vi "Server_Main Stop.vi"(8 "error in":errorcluster) -> (0 "error out":errorcluster)   [LabVIEW 2018, in "Cloud Server.lvlib"]
uses:
  Cloud Server.lvlib
  Data Def/Server_Main Loop Queue Data.ctl
  Data Def/Server_Main Loop State.ctl
  Data Def/Server_Server Write Queue Data.ctl
  Data Def/Server_FGV Method.ctl
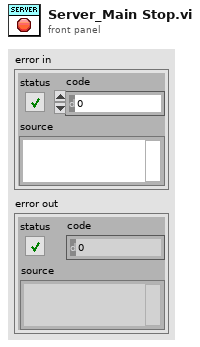
[diagram p1: front panel]
types:
  T1 = typedef "Cloud Server.lvlib/Server_Server Write Queue Data.ctl" = cluster{"connection ID":refnum<k5>, "Meta Data":string, "Data":variant}
  T2 = typedef "Cloud Server.lvlib/Server_Main Loop Queue Data.ctl" = cluster{"Main Loop State":T3, "Data":variant}
  T3 = typedef "Cloud Server.lvlib/Server_Main Loop State.ctl" = enum16{"Detect", "Save", "Training", "Refresh User Name", "Stop"}
  T4 = typedef "Cloud Server.lvlib/Server_FGV Method.ctl" = enum16{"Get", "Put"}
  T5 = typedef "Cloud Server.lvlib/Server_Main Data.ctl" = cluster{"Main VI Ref.":refnum<vi>, "Listener ID":refnum<k5>, "Meta data":T6[], "Main Queue":T8, "User Picture":T9}
  T6 = typedef "stm_MetaElement.ctl" = cluster{"Name":T7}
  T7 = typedef "stm_MetaDataElement.ctl" = string
  T8 = typedef "Cloud Server.lvlib/Server_Main Queue.ctl" = cluster{"Server Write Queue":refnum<queue>, "Main Loop Queue":refnum<queue>}
  T9 = typedef "IMAQ Image.ctl" = refnum<image>
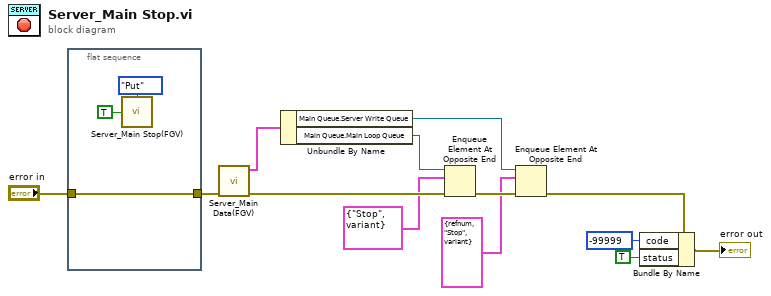
[diagram p0: block diagram]
diagram:
  n1 = flat-sequence {
    tunnel: "error in" -> [w14]
    tunnel: [w14] -> w12
    frame #0 {
      n2 = call "Server_Main Stop(FGV).vi"("FGV Method"=Server_FGV_Method."Put", "Stop In"=TRUE) -> ()  [unwired: 2 in, 1 out]
    }
  }
  n3 = call "Server_Main Data(FGV).vi"("error in"=w12) -> ("error out"=w10:errorcluster, "Main Data Out"=w11:T5)  [unwired: 9 in]
  n4 = Unbundle By Name(w11) -> ("Main Queue.Server Write Queue"=w6:refnum<queue>, "Main Queue.Main Loop Queue"=w9:refnum<queue>)
  n5 = Enqueue Element At Opposite End(queue=w9, element=T2 {"Main Loop State"=enum."Stop", "Data"=variant}, error in (no error)=w10) -> (error out=w7:errorcluster)  [unwired: 1 in, 2 out]
  n6 = Enqueue Element At Opposite End(queue=w6, element=T1 {"connection ID"=refnum, "Meta Data"="Stop", "Data"=variant}, error in (no error)=w7) -> (error out=w2:errorcluster)  [unwired: 1 in, 2 out]
  n7 = Bundle By Name(cluster=w2, "code"=-99999, "status"=TRUE) -> (→"error out":errorcluster)
